vi "Elevator Test.vi"() -> (1 "Error Debug":string, 2 "Error Source":string)   [LabVIEW 2018]
uses:
  Elevator/Implementation/Infrastructure/Positions.ctl
  <extravilib>/ChannelInstances/Event Messenger-t'Command Status Info.ctl'.lvlib
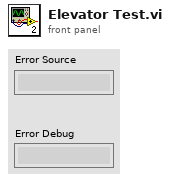
[diagram p1: front panel]
types:
  T1 = typedef "Positions.ctl" = enum16{"MANUAL", "Bottom (intake, etc)", "Lower Hold"}
  T2 = typedef "Command Status Info.ctl" = cluster{"Name":string, "Status":T3, "notifier out":T4}
  T3 = typedef "Completion Status.ctl" = enum16{"Successful", "Aborted", "Incomplete"}
  T4 = typedef "Completion Notifier.ctl" = refnum<notifier>
  T5 = typedef "Event Messenger-t'Command Status Info.ctl'.lvlib/))Channel.ctl" = refnum<queue>
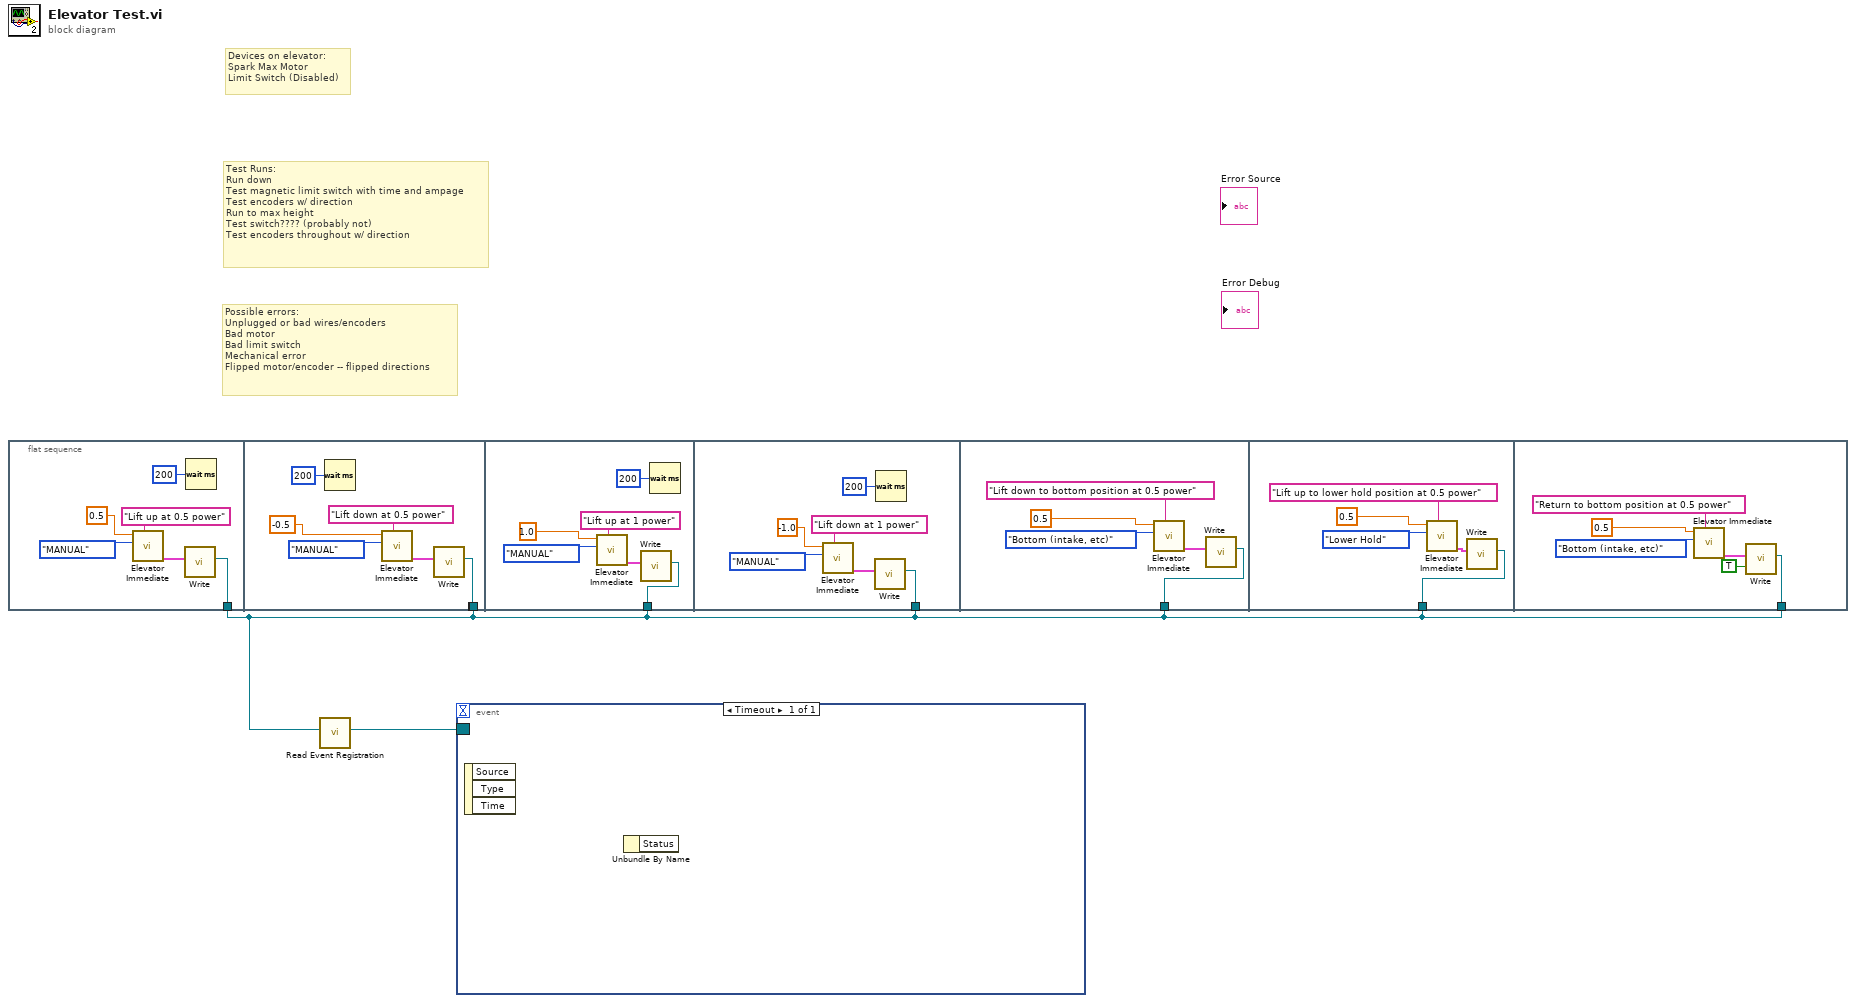
[diagram p0: block diagram]
diagram:
  # "Devices on elevator:\nSpark Max Motor\nLimit Switch (Disabled)"
  # "Possible errors:\nUnplugged or bad wires/encoders\nBad motor\nBad limit switch\nMechanical error\nFlipped motor/encoder -- flipped directions"
  # "Test Runs:\nRun down\nTest magnetic limit switch with time and ampage\nTest encoders w/ direction\nRun to max height\nTest switch???? (probably not)\nTest encoders throughout w/ direction"
  n1 = flat-sequence {
    tunnel: [w3] -> w2
    tunnel: [w9] -> _
    tunnel: w2 -> [_]
    tunnel: w2 -> [w15]
    tunnel: w2 -> [w21]
    tunnel: w2 -> [w27]
    tunnel: w2 -> [w32]
    tunnel: w2 -> [w38]
    frame #0 {
      n2 = call "Elevator Immediate.vi"("Description"="Lift up at 0.5 power", "Position"=Positions."MANUAL", "Setpoint"=0.5) -> ("Command Info Out"=w5:T2)  [unwired: 8 in]
      n3 = call <extravilib>:"Write.vi"("element"=w5) -> ("channel"=w3:T5)  [unwired: 9 in, 1 out]
      n4 = Wait (ms)(milliseconds to wait=u32 200) -> ()  [unwired: 1 out]
    }
    frame #1 {
      n5 = Wait (ms)(milliseconds to wait=u32 200) -> ()  [unwired: 1 out]
      n6 = call "Elevator Immediate.vi"("Description"="Lift down at 0.5 power", "Position"=Positions."MANUAL", "Setpoint"=-0.5) -> ("Command Info Out"=w11:T2)  [unwired: 8 in]
      n7 = call <extravilib>:"Write.vi"("element"=w11) -> ("channel"=w9:T5)  [unwired: 9 in, 1 out]
    }
    frame #2 {
      n8 = call "Elevator Immediate.vi"("Description"="Lift up at 1 power", "Position"=Positions."MANUAL", "Setpoint"=1.0) -> ("Command Info Out"=w16:T2)  [unwired: 8 in]
      n9 = call <extravilib>:"Write.vi"("element"=w16) -> ("channel"=w15:T5)  [unwired: 9 in, 1 out]
      n10 = Wait (ms)(milliseconds to wait=u32 200) -> ()  [unwired: 1 out]
    }
    frame #3 {
      n11 = call "Elevator Immediate.vi"("Description"="Lift down at 1 power", "Position"=Positions."MANUAL", "Setpoint"=-1.0) -> ("Command Info Out"=w22:T2)  [unwired: 8 in]
      n12 = call <extravilib>:"Write.vi"("element"=w22) -> ("channel"=w21:T5)  [unwired: 9 in, 1 out]
      n13 = Wait (ms)(milliseconds to wait=u32 200) -> ()  [unwired: 1 out]
    }
    frame #4 {
      n14 = call "Elevator Immediate.vi"("Description"="Lift down to bottom position at 0.5 power", "Position"=Positions."Bottom (intake, etc)", "Setpoint"=0.5) -> ("Command Info Out"=w28:T2)  [unwired: 8 in]
      n15 = call <extravilib>:"Write.vi"("element"=w28) -> ("channel"=w27:T5)  [unwired: 9 in, 1 out]
    }
    frame #5 {
      n16 = call "Elevator Immediate.vi"("Description"="Lift up to lower hold position at 0.5 power", "Position"=Positions."Lower Hold", "Setpoint"=0.5) -> ("Command Info Out"=w33:T2)  [unwired: 8 in]
      n17 = call <extravilib>:"Write.vi"("element"=w33) -> ("channel"=w32:T5)  [unwired: 9 in, 1 out]
    }
    frame #6 {
      n18 = call "Elevator Immediate.vi"("Description"="Return to bottom position at 0.5 power", "Position"=Positions."Bottom (intake, etc)", "Setpoint"=0.5) -> ("Command Info Out"=w39:T2)  [unwired: 8 in]
      n19 = call <extravilib>:"Write.vi"("last element? (F)"=TRUE, "element"=w39) -> ("channel"=w38:T5)  [unwired: 8 in, 1 out]
    }
  }
  n20 = call <extravilib>:"Read Event Registration.vi"("channel"=w2) -> ("event registration refnum"=w1:refnum<event-registration>)  [unwired: 10 in]
  n21 = event shown="[0] Timeout" {
    selector: w1 -> [_]
    dyn-events: _ -> [_]
    timeout: _ -> [_]
    event Timeout {
      n22 = event-data() -> ()  [unwired: 1 in, 3 out]
      n23 = Unbundle By Name() -> ()  [unwired: 1 in, 1 out]
    }
  }
